vi "MicCalib.vi"() -> ()   [LabVIEW 2017]
doc: "This example demonstrates how to acquire a single buffer of voltage measurements using a DAQmx device.\n\nFor instructions on how to connect your signals to the DAQ device, refer to your device documentation."
uses:
  <vilib>/Utility/error.llb/DialogType.ctl
  <vilib>/DAQmx/read.llb/DAQmx Read (Analog 1D Wfm NChan NSamp).vi
  <vilib>/Analysis/baseanly.llb/Scale 1D.vi
  <vilib>/DAQmx/create/channels.llb/DAQmx Create Channel (AI-Voltage-Basic).vi
  <vilib>/DAQmx/configure/timing.llb/DAQmx Timing (Sample Clock).vi
  <vilib>/DAQmx/configure/task.llb/DAQmx Configure Logging (TDMS).vi
  <vilib>/DAQmx/configure/trigger.llb/DAQmx Start Trigger (Digital Edge).vi
  <vilib>/DAQmx/configure/trigger.llb/DAQmx Start Trigger (Time).vi
  <vilib>/DAQmx/configure/trigger.llb/DAQmx Start Trigger (Analog Edge).vi
  <vilib>/DAQmx/configure/trigger.llb/DAQmx Reference Trigger (Digital Edge).vi
  <vilib>/DAQmx/configure/trigger.llb/DAQmx Reference Trigger (Analog Edge).vi
  <vilib>/DAQmx/miscellaneous.llb/DAQmx Fill In Error Info.vi
  <vilib>/measure/madcrms.llb/Basic Averaged DC-RMS for N Chan.vi
  <vilib>/measure/madcrms.llb/Averaged DC-RMS for N Chan.vi
  <resource>/objmgr/daqmx.rc
  <vilib>/measure/NI_MAPro.lvlib
  <vilib>/Analysis/NI_AALBase.lvlib
panel:
  out "V rms":dbl[](array[numeric]) format="%.2p"
  out "RMS value waveforms":waveform(dbl)[](array[waveform])
  in  "Trigger Type":T1(tab)
  in  "Digital Start Trigger Edge":i32(ring)=10280 caption="Edge" items=["Rising"=10280, "Falling"=10171]
  in  "Digital Start Trigger Source":tag="/Dev1/PFI0" caption="Source"
  in  "Digital Pause Trigger Pause When":i32(ring)=10192 caption="Pause When" items=["High"=10192, "Low"=10214]
  in  "Digital Pause Trigger Source":tag="/Dev1/PFI0" caption="Source"
  in  "Digital Reference Trigger Source":tag="/Dev1/PFI0" caption="Source"
  in  "Digital Reference Trigger Edge":i32(ring)=10280 caption="Edge" items=["Rising"=10280, "Falling"=10171]
  in  "Digital Reference Pretrigger Samples":u32 caption="Pretrigger Samples"
  in  "Analog Start Trigger Level":dbl caption="Level" format="%0.2f"
  in  "Analog Start Trigger Hysteresis":dbl caption="Hysteresis" format="%.2f"
  in  "Analog Start Trigger Slope":i32(ring)=10280 caption="Slope" items=["Rising"=10280, "Falling"=10171]
  in  "Analog Start Trigger Source":string="APFI0" caption="Source"
  in  "Analog Pause Trigger Source":string="APFI0" caption="Source"
  in  "Analog Pause Trigger Pause When":i32(ring)=10093 caption="Pause When" items=["Above Level"=10093, "Below Level"=10107]
  in  "Analog Pause Trigger Level":dbl caption="Level" format="%.2f"
  in  "Analog Reference Trigger Source":string="APFI0" caption="Source"
  in  "Analog Reference Trigger Level":dbl caption="Level" format="%.2f"
  in  "Analog Reference Trigger Slope":i32(ring)=10280 caption="Slope" items=["Rising"=10280, "Falling"=10171]
  in  "Analog Reference Pretrigger Samples":u32 caption="Pretrigger Samples"
  in  "When":timestamp
  in  "Select Time\nManually":bool
  out "Waveform Graph":waveform(dbl)[](graph)
  in  "TDMS File Path":path
  in  "Number of Samples":i32=512000
  in  "Sample Rate":dbl=51200.0
  in  "Sample Clock Source":tag="OnboardClock"
  in  "Terminal Configuration":i32(ring)=-1 items=["default"=-1, "RSE"=10083, "NRSE"=10078, "Differential"=10106, "Pseudodifferential"=12529]
  in  "Max Voltage":dbl=5.0
  in  "Min Voltage":dbl=-5.0
  in  "Physical Channel":tag="cDAQ1Mod1/ai0"
  out "Actual Sample Rate":dbl format="%0.2f"
  in  "Logging Mode":i32(ring)=10231 items=["Off"=10231, "Log and Read"=15842]
  # "Channel Settings"
  # "Acquired Data"
  # "Timing Settings"
  # "Trigger Settings"
  # "Logging Settings"
  # "To enable triggers, select a tab above, and configure the settings.\n\nNot all hardware supports all trigger types. Refer to your device documentation for more information."
  # "If time is not manually set, task will begin after 10 seconds"
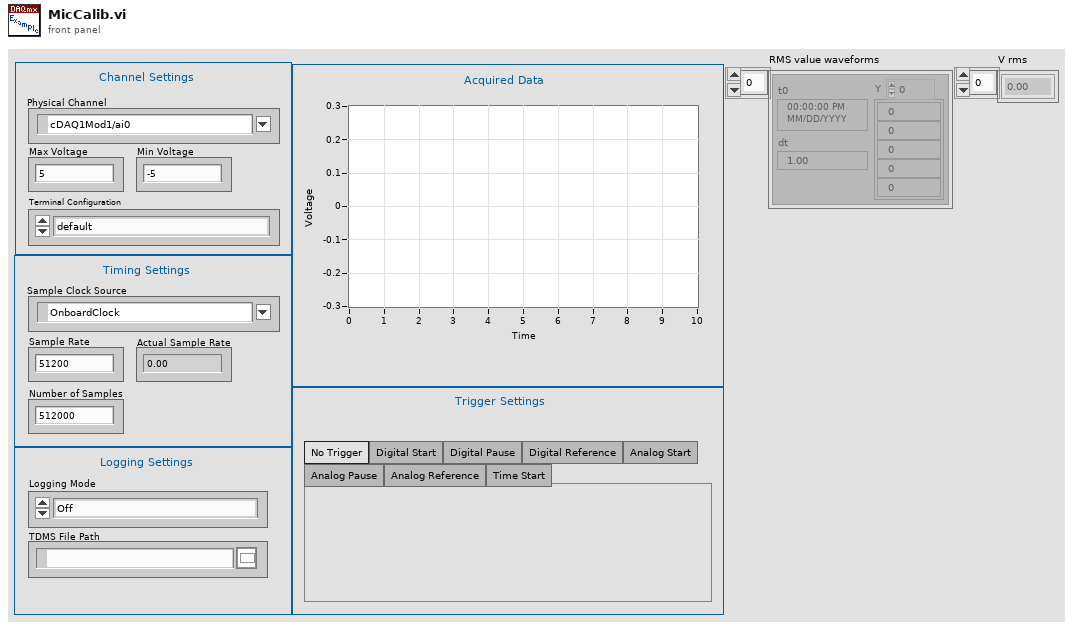
[diagram p1: front panel]
types:
  T1 = enum32{"No Trigger", "Digital Start", "Digital Pause", "Digital Reference", "Analog Start", "Analog Pause", "Analog Reference", "Time Start"}
  T2 = typedef "DialogType.ctl" = u16
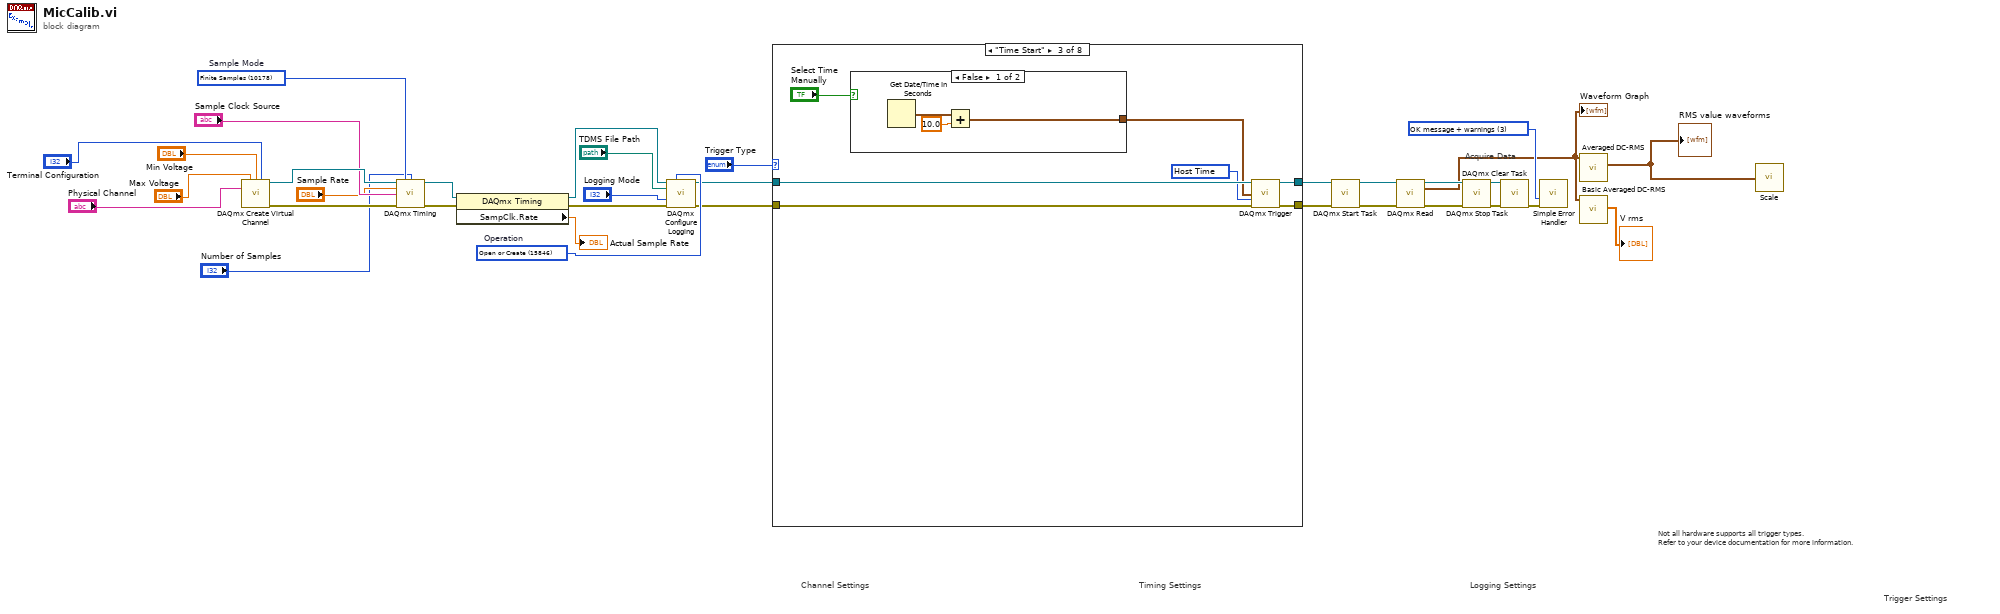
[diagram p0: block diagram]
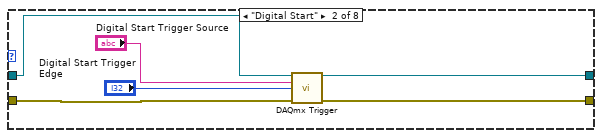
[diagram p3: hidden frame]
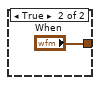
[diagram p4: hidden frame]
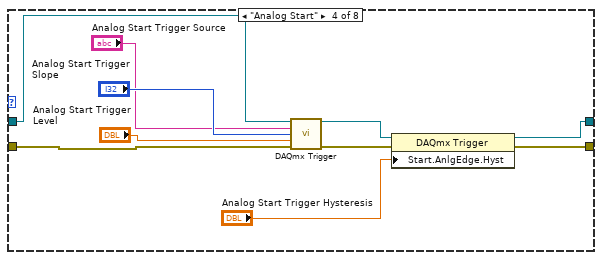
[diagram p5: hidden frame]
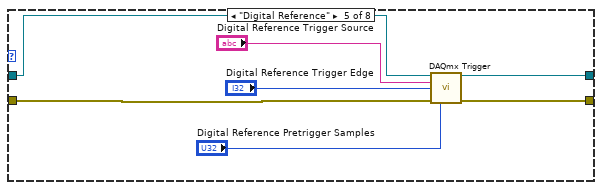
[diagram p6: hidden frame]
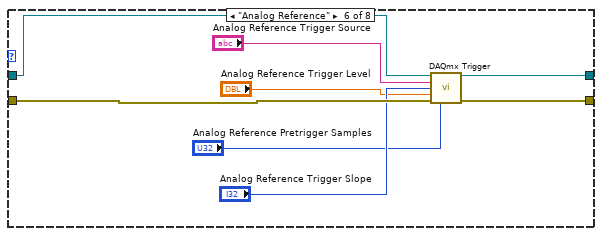
[diagram p7: hidden frame]
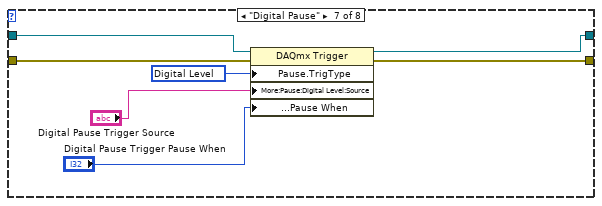
[diagram p8: hidden frame]
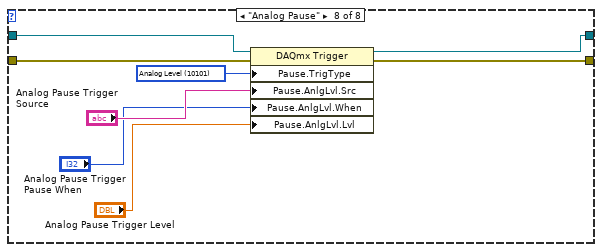
[diagram p9: hidden frame]
diagram:
  w9 = T2 3 items=["no dialog", "OK message", "continue or stop message", "OK message + warnings", "continue/stop + warnings"] ("type of dialog (OK msg:1)")
  w27 = 15846 items=["Open"=10437, "Open or Create"=15846, "Create or Replace"=15847, "Create"=15848]  # Operation
  w32 = 10178 items=["Finite Samples"=10178, "Continuous Samples"=10123, "Hardware Timed Single Point"=12522]  # Sample Mode
  # "Not all hardware supports all trigger types.\nRefer to your device documentation for more information."
  # "Trigger Settings"
  # "Acquire Data"
  # "Timing Settings"
  # "Channel Settings"
  # "Logging Settings"
  n1 = call-poly <vilib>:"DAQmx Create Virtual Channel.vi"("maximum value"="Max Voltage", "minimum value"="Min Voltage", "input terminal configuration"="Terminal Configuration", "physical channels"="Physical Channel") -> ("task out"=w30:refnum<k21>, "error out"=w31:errorcluster)  [unwired: 10 in]
  n2 = call-poly <vilib>:"DAQmx Timing.vi"("task/channels in"=w30, "sample mode"=w32, "samples per channel"="Number of Samples", "rate"="Sample Rate", "source"="Sample Clock Source", "error in"=w31) -> ("task out"=w34:refnum<k21>, "error out"=w33:errorcluster)  [unwired: 8 in]
  n3 = property class="DAQmx Timing"(reference=w34, error in=w33) -> (reference out=w29:refnum<k21>, error out=w28:errorcluster, "SampClk.Rate"=→"Actual Sample Rate":dbl)
  n4 = call-poly <vilib>:"DAQmx Configure Logging.vi"("task/channels in"=w29, "operation"=w27, "file path"="TDMS File Path", "logging mode"="Logging Mode", "error in"=w28) -> ("task out"=w7:refnum<k21>, "error out"=w6:errorcluster)  [unwired: 9 in]
  n5 = case shown="\"Time Start\"" "Trigger Type" {
    tunnel: w7 -> [w36 w42 w49 w63 w70 w78 w85 w93]
    tunnel: w6 -> [w35 w41 w48 w62 w69 w77 w82 w90]
    tunnel: [w36 w40 w47 w60 w68 w76 w84 w92] -> w5
    tunnel: [w35 w39 w46 w59 w67 w75 w83 w91] -> w4
    frame "No Trigger", Default {
    }
    frame "Digital Start" {
      n6 = call-poly <vilib>:"DAQmx Trigger.vi"("task/channels in"=w42, "source"="Digital Start Trigger Source", "edge"="Digital Start Trigger Edge", "error in"=w41) -> ("task out"=w40:refnum<k21>, "error out"=w39:errorcluster)  [unwired: 10 in]
    }
    frame "Time Start" {
      w45 = 16126 items=["Host Time"=16126, "I/O Device Time"=16127] ("timescale")
      n7 = case shown="False" "Select Time\nManually" {
        tunnel: [w51 "When"] -> w43
        frame False {
          n8 = Get Date/Time In Seconds() -> (seconds since 1Jan1904=w52:timestamp)
          n9 = Add(x=w52, y=10.0) -> (x+y=w51:timestamp)
        }
        frame True {
        }
      }
      n10 = call-poly <vilib>:"DAQmx Trigger.vi"("task/channels in"=w49, "when"=w43, "timescale"=w45, "error in"=w48) -> ("task out"=w47:refnum<k21>, "error out"=w46:errorcluster)  [unwired: 10 in]
    }
    frame "Analog Start" {
      n11 = call-poly <vilib>:"DAQmx Trigger.vi"("task/channels in"=w63, "source"="Analog Start Trigger Source", "slope"="Analog Start Trigger Slope", "level"="Analog Start Trigger Level", "error in"=w62) -> ("task out"=w58:refnum<k21>, "error out"=w57:errorcluster)  [unwired: 9 in]
      n12 = property class="DAQmx Trigger"(reference=w58, error in=w57, "Start.AnlgEdge.Hyst"="Analog Start Trigger Hysteresis") -> (reference out=w60:refnum<k21>, error out=w59:errorcluster)
    }
    frame "Digital Reference" {
      n13 = call-poly <vilib>:"DAQmx Trigger.vi"("task/channels in"=w70, "source"="Digital Reference Trigger Source", "edge"="Digital Reference Trigger Edge", "error in"=w69, "pretrigger samples per channel"="Digital Reference Pretrigger Samples") -> ("task out"=w68:refnum<k21>, "error out"=w67:errorcluster)  [unwired: 9 in]
    }
    frame "Analog Reference" {
      n14 = call-poly <vilib>:"DAQmx Trigger.vi"("task/channels in"=w78, "source"="Analog Reference Trigger Source", "slope"="Analog Reference Trigger Slope", "level"="Analog Reference Trigger Level", "error in"=w77, "pretrigger samples per channel"="Analog Reference Pretrigger Samples") -> ("task out"=w76:refnum<k21>, "error out"=w75:errorcluster)  [unwired: 8 in]
    }
    frame "Digital Pause" {
      w81 = 10152 items=["Analog Level"=10101, "Analog Window"=10103, "Digital Level"=10152, "Digital Pattern"=10398, "None"=10230] ("Pause.TrigType")
      n15 = property class="DAQmx Trigger"(reference=w85, error in=w82, "Pause.TrigType"=w81, "More:Pause:Digital Level:Source"="Digital Pause Trigger Source", "More:Pause:Digital Level:Pause When"="Digital Pause Trigger Pause When") -> (reference out=w84:refnum<k21>, error out=w83:errorcluster)
    }
    frame "Analog Pause" {
      w89 = 10101 items=["Analog Level"=10101, "Analog Window"=10103, "Digital Level"=10152, "Digital Pattern"=10398, "None"=10230] ("Pause.TrigType")
      n16 = property class="DAQmx Trigger"(reference=w93, error in=w90, "Pause.TrigType"=w89, "Pause.AnlgLvl.Src"="Analog Pause Trigger Source", "Pause.AnlgLvl.When"="Analog Pause Trigger Pause When", "Pause.AnlgLvl.Lvl"="Analog Pause Trigger Level") -> (reference out=w92:refnum<k21>, error out=w91:errorcluster)
    }
  }
  n17 = call <vilib>:"DAQmx Start Task.vi"("task/channels in"=w5, "error in"=w4) -> ("task out"=w26:refnum<k21>, "error out"=w25:errorcluster)  [unwired: 12 in]
  n18 = call-poly <vilib>:"DAQmx Read.vi"("task/channels in"=w26, "error in"=w25) -> ("task out"=w11:refnum<k21>, "data"=w3:waveform(dbl)[], "error out"=w10:errorcluster)  [unwired: 11 in]
  "Waveform Graph" <- w3
  n19 = call <vilib>:"DAQmx Stop Task.vi"("task/channels in"=w11, "error in"=w10) -> ("task out"=w13:refnum<k21>, "error out"=w12:errorcluster)  [unwired: 12 in]
  n20 = call <vilib>:"DAQmx Clear Task.vi"("task in"=w13, "error in"=w12) -> ("error out"=w24:errorcluster)  [unwired: 13 in]
  n21 = call <vilib>:"Simple Error Handler.vi"("type of dialog (OK msg:1)"=w9, "error in (no error)"=w24) -> ()  [unwired: 3 in, 5 out]
  n22 = call-poly <vilib>:"Averaged DC-RMS.vi"("signals in"=w3) -> ("RMS value waveforms"=w1:waveform(dbl)[])  [unwired: 6 in, 4 out]
  "RMS value waveforms" <- w1
  n23 = call-poly <vilib>:"Basic Averaged DC-RMS.vi"("signals in"=w3) -> ("RMS values"=→"V rms":dbl[])  [unwired: 7 in, 3 out]
  n24 = call-poly <vilib>:"Scale.vi"("X"=w1) -> ()  [unwired: 4 out]
